vi "test_Get Bitfile Scalars_Error.vi"(8 "error in (no error)":errorcluster, 11 "TestCase in":refnum<class "FPGA Addon Scripting API Unit Tests.lvclass">=refnum) -> (0 "error out":errorcluster, 3 "TestCase out":refnum<class "FPGA Addon Scripting API Unit Tests.lvclass">)   [LabVIEW 2026, in "FPGA Addon Scripting API Unit Tests.lvclass"]
uses:
  FPGA Addon Scripting API Unit Tests.lvclass
  FPGA Addon Test Class/FPGA Addon Test Class.lvclass
  APIs/Scripting API/Scripting API.lvlib
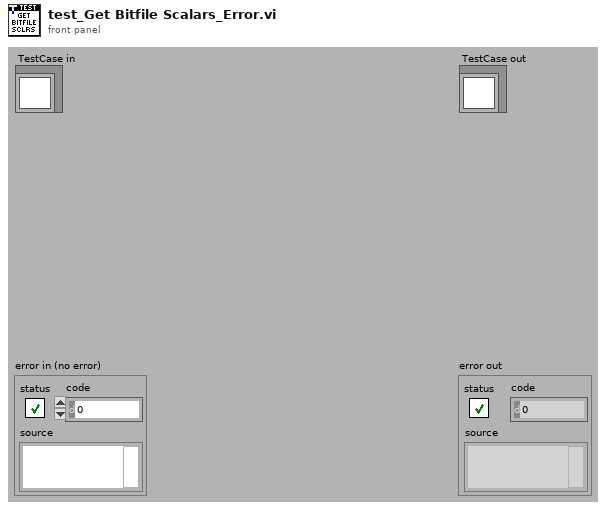
[diagram p1: front panel]
types:
  T1 = typedef "Custom Device API.lvlib/Custom Device Item Ref.ctl" = u64
  T2 = typedef "Scripting API.lvlib/Output Scalar Data.ctl" = cluster{"Bitfile Name":string, "SysDef Channel Name":string, "Imported":bool, "Data Type":T3}
  T3 = typedef "FPGA Addon Shared.lvlib/FPGA Addon Data Type.ctl" = enum8{"<Null>", "I8", "I16", "I32", "I64", "U8", "U16", "U32", "U64", "SGL", "Boolean", "Analog PWM In Settings", "Analog PWM In", "Digital PWM In Settings", "Digital PWM In", "Digital PWM Out", "Sine Out", "FXP", "FXP+/-24.5", "FXP+/-16.5", "FXP+/-32.8", "FXP+/-64.32", "FXP+/-16.7", "FXP+/-20.5", "FXP+/-27.5", "FXP+/-32.16", "FXP+16.3", "FXP+18.3", "Digital Static In", "Digital Static Out", "Digital Static In Settings", "Digital WSS Out", "Quad Encoder Settings", "Quad Encoder In", "Group"}
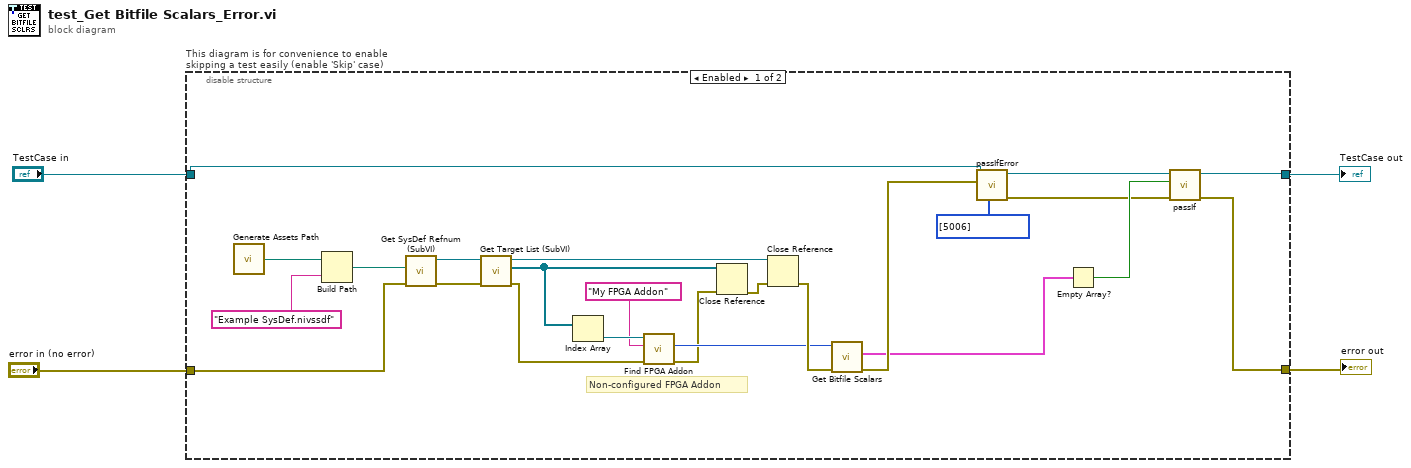
[diagram p0: block diagram]
diagram:
  n1 = disable-structure "This diagram is for convenience to enable skipping a test easily (enable 'Skip' case)" shown="Enabled" {
    disable-tunnel: "TestCase in" -> [w13 w32]
    disable-tunnel: [w5 w30] -> w1
    disable-tunnel: [w6 w31] -> w3
    disable-tunnel: "error in (no error)" -> [w24 w29]
    frame Enabled {
      # "Non-configured FPGA Addon"
      n2 = call "Generate Assets Path.vi"() -> ("Assets path"=w28:path)
      n3 = Build Path(base path=w28, name or relative path="Example SysDef.nivssdf") -> (appended path=w26:path)
      n4 = call "Get SysDef Refnum (SubVI).vi"("error in (no error)"=w24, "System Definition path"=w26) -> ("error out"=w23:errorcluster, "NationalInstruments.VeriStand.SystemDefinitionAPI.SystemDefinition"=w25:refnum<k39>)  [unwired: 8 in]
      n5 = call "Get Target List (SubVI).vi"("error in (no error)"=w23, "NationalInstruments.VeriStand.SystemDefinitionAPI.SystemDefinition"=w25) -> ("error out"=w18:errorcluster, "Target List Refnums"=w22:refnum<k39>[], "NationalInstruments.VeriStand.SystemDefinitionAPI.SystemDefinition"=w21:refnum<k39>)  [unwired: 7 in]
      n6 = Index Array(array=w22) -> (element=w19:refnum<k39>)  [unwired: 1 in]
      n7 = call "Find FPGA Addon.vi"("error in"=w18, "FPGA addon name"="My FPGA Addon", "NationalInstruments.VeriStand.SystemDefinitionAPI.Target"=w19) -> ("error out"=w14:errorcluster, "FPGA addon refnum out"=w15:T1)  [unwired: 5 in, 2 out]
      n8 = Close Reference(reference=w22, error in (no error)=w14) -> (error out=w20:errorcluster)
      n9 = Close Reference(reference=w21, error in (no error)=w20) -> (error out=w16:errorcluster)
      n10 = call "Get Bitfile Scalars.vi"("error in"=w16, "FPGA addon refnum in"=w15) -> ("error out"=w12:errorcluster, "bitfile scalars out"=w10:T2[])  [unwired: 7 in, 1 out]
      n11 = call-dynamic "passIfError.vi"("passing error codes (default = any error code)"=i32[] [5006], "error"=w12, "TestCase in"=w13) -> ("error out"=w7:errorcluster, "TestCase out"=w8:refnum<class "FPGA Addon Scripting API Unit Tests.lvclass">)  [unwired: 7 in]
      n12 = Empty Array?(array=w10) -> (empty?=w9:bool)
      n13 = call-dynamic "passIf.vi"("error in (no error)"=w7, "pass"=w9, "TestCase in"=w8) -> ("error out"=w6:errorcluster, "TestCase out"=w5:refnum<class "FPGA Addon Scripting API Unit Tests.lvclass">)  [unwired: 7 in]
    }
    frame Disabled {
      # "skip test result while test is under development"
      n14 = call <vilib>:"skip.vi"("error in (no error)"=w29, "TestCase in"=w32) -> ("error out"=w31:errorcluster, "TestCase out"=w30:refnum<class "FPGA Addon Scripting API Unit Tests.lvclass">)  [unwired: 8 in]
    }
  }
  "error out" <- w3
  "TestCase out" <- w1
